vi "Configure Output Range.vi"(0 "VISA resource name":refnum<visa-resource-name>, 5 "Channel Select":enum16{"Channel 1", "Channel 2", "Channel 3"}(ring), 7 "MAX Voltage Limit":dbl format="%_6g", 9 "Enable Max. Voltage (T: Enable)":bool=TRUE, 11 "error in (no error)":errorcluster) -> (4 "VISA resource name out":refnum<visa-resource-name>, 15 "error out":errorcluster)   [LabVIEW 2018, in "Keithley KE22xx Series.lvlib"]
doc: "Configure the Maximum range for Voltage function of specified channel.\n\nNote: Call the Enable Output.vi before Configure Output Range.vi"
uses:
  Keithley KE22xx Series.lvlib
panel:
  # "© 2012 Keithley Instruments, Inc. ALL RIGHTS RESERVED"
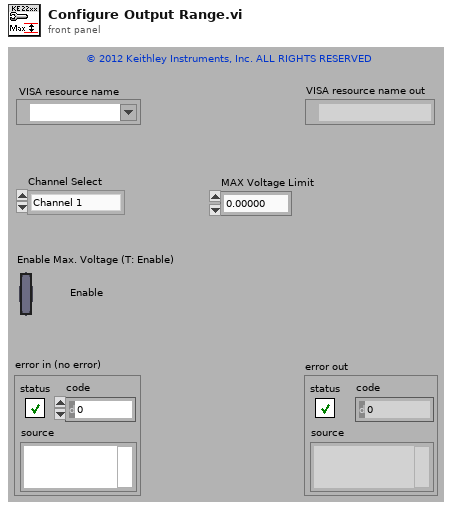
[diagram p1: front panel]
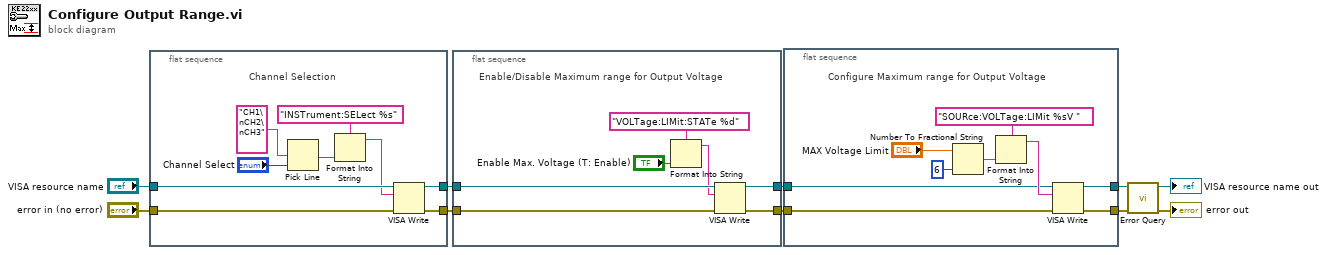
[diagram p0: block diagram]
diagram:
  n1 = flat-sequence {
    tunnel: "VISA resource name" -> [w18]
    tunnel: "error in (no error)" -> [w17]
    tunnel: [w12] -> w4
    tunnel: [w11] -> w2
    frame #0 {
      # "Channel Selection"
      n2 = Pick Line(multi-line string="CH1\nCH2\nCH3", line index="Channel Select") -> (output string=w13:string)  [unwired: 1 in]
      n3 = Format Into String(format string="INSTrument:SELect %s", w13) -> (resulting string=w16:string)  [unwired: 2 in, 1 out]
      n4 = VISA Write(VISA resource name=w18, write buffer=w16, error in (no error)=w17) -> (VISA resource name out=w12:refnum<visa-resource-name>, error out=w11:errorcluster)  [unwired: 1 out]
    }
  }
  n5 = flat-sequence {
    tunnel: w4 -> [w26]
    tunnel: [w25] -> w3
    tunnel: w2 -> [w24]
    tunnel: [w23] -> w1
    frame #0 {
      # "Enable/Disable Maximum range for Output Voltage"
      n6 = Format Into String(format string="VOLTage:LIMit:STATe %d", "Enable Max. Voltage (T: Enable)") -> (resulting string=w20:string)  [unwired: 2 in, 1 out]
      n7 = VISA Write(VISA resource name=w26, write buffer=w20, error in (no error)=w24) -> (VISA resource name out=w25:refnum<visa-resource-name>, error out=w23:errorcluster)  [unwired: 1 out]
    }
  }
  n8 = flat-sequence {
    tunnel: [w31] -> w6
    tunnel: [w30] -> w5
    tunnel: w3 -> [w29]
    tunnel: w1 -> [w28]
    frame #0 {
      # "Configure Maximum range for Output Voltage"
      n9 = Number To Fractional String(number="MAX Voltage Limit", precision (6)=i16 6) -> (F-format string=w32:string)  [unwired: 2 in]
      n10 = Format Into String(format string="SOURce:VOLTage:LIMit %sV ", w32) -> (resulting string=w35:string)  [unwired: 2 in, 1 out]
      n11 = VISA Write(VISA resource name=w29, write buffer=w35, error in (no error)=w28) -> (VISA resource name out=w31:refnum<visa-resource-name>, error out=w30:errorcluster)  [unwired: 1 out]
    }
  }
  n12 = call "Error Query.vi"("error in (no error)"=w5, "VISA resource name"=w6) -> ("error out"=→"error out":errorcluster, "VISA resource name out"=→"VISA resource name out":refnum<visa-resource-name>)  [unwired: 6 in, 2 out]
